vi "PH_BlackBox.PC Write PSDB.vi"(0 "i ref in":refnum<vi>, 5 "error IO":errorcluster) -> (14 "i ref out":refnum<vi>, 19 "error out":errorcluster)   [LabVIEW 2014, in "PH_BlackBox.lvlib"]
doc: "This is the proc case which writes data to the PHELIX shot data base."
uses:
  PH_BlackBox.lvlib
  PH_Basics/PH_PSDBWriter/PH_PSDBWriter.lvlib
  PH_Basics/PH_StatusHandler/PH_StatusHandler.lvlib
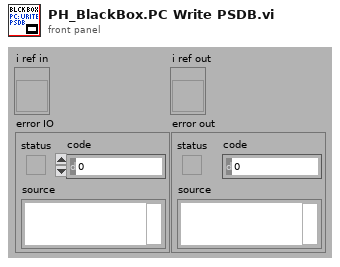
[diagram p1: front panel]
types:
  T1 = typedef "PH_BlackBox.lvlib/PH_BlackBox.i attribute.ctl" = cluster{"BB Remote Controlled?":bool, "GUI Refs":T2, "Position IN":T3, "Position OUT":T3, "BB Remote Controlled by other Instance?":bool, "Recipient":string, "Number":i32, "Caption Move":string, "Caption Out":string, "Caption In":string}
  T2 = typedef "PH_BlackBox.lvlib/PH_BlackBox.GUI Refs.ctl" = cluster{"MOVE IN":refnum<vi>, "MOVE":refnum<vi>, "IN":refnum<vi>, "OUT":refnum<vi>, "REMOTE":refnum<vi>, "GUI-Knob Move":refnum<vi>, "GUI-Knob Move in":refnum<vi>, "POWER ON":refnum<vi>, "Delete":refnum<vi>, "Function Textfield":refnum<vi>}
  T3 = typedef "PH_StatusHandler.lvlib/PH_StatusHandler.Status.ctl" = i16
  T4 = typedef "PH_PSDBWriter.lvlib/PH_PSDBWriter.String dataset.ctl" = cluster{"name":string, "data":string, "unit":string}
  T5 = typedef "PH_PSDBWriter.lvlib/PH_PSDBWriter.PSDB Dataset.ctl" = cluster{"Version":i32, "2D data Input":T6[], "Boolean Input":T8[], "Image Input":T9[], "Numeric Input":T11[], "String Input":T4[]}
  T6 = typedef "PH_PSDBWriter.lvlib/PH_PSDBWriter.2D dataset.ctl" = cluster{"name":string, "data":dbl[][], "axis description":T7}
  T7 = typedef "PSDB.lvlib/PSDB_AxisDescription.ctl" = cluster{"x axis label":string, "y axis label":string, "x axis unit":string, "y axis unit":string}
  T8 = typedef "PH_PSDBWriter.lvlib/PH_PSDBWriter.Boolean dataset.ctl" = cluster{"name":string, "data":bool, "unit":string}
  T9 = typedef "PH_PSDBWriter.lvlib/PH_PSDBWriter.Image dataset.ctl" = cluster{"name":string, "data":T10, "unit":string}
  T10 = typedef "IMAQ Image.ctl" = refnum<image>
  T11 = typedef "PH_PSDBWriter.lvlib/PH_PSDBWriter.Numeric dataset.ctl" = cluster{"name":string, "data":dbl, "unit":string}
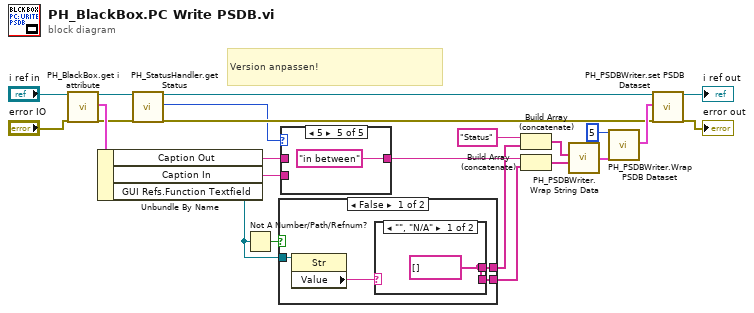
[diagram p0: block diagram]
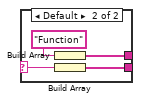
[diagram p2: hidden frame]
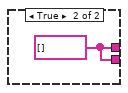
[diagram p3: hidden frame]
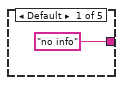
[diagram p4: hidden frame]
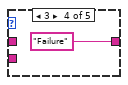
[diagram p7: hidden frame]
diagram:
  # "Version anpassen!"
  n1 = call "PH_BlackBox.get i attribute.vi"("i ref in"="i ref in", "error in (no error)"="error IO") -> ("i ref out"=w3:refnum<vi>, "i attribute"=w23:T1, "error out"=w22:errorcluster)  [unwired: 15 in]
  n2 = Unbundle By Name(w23) -> ("Caption Out"=w12:string, "Caption In"=w11:string, "GUI Refs.Function Textfield"=w7:refnum<vi>)
  n3 = call "PH_StatusHandler.get Status.vi"("VI in"=w3, "error in"=w22) -> ("VI out"=w2:refnum<vi>, "Status"=w1:T3, "error out"=w4:errorcluster)  [unwired: 15 in]
  n4 = Not A Number/Path/Refnum?(number/path/refnum=w7) -> (NaN/Path/Refnum?=w8:bool)
  n5 = case shown="False" w8 {
    tunnel: w7 -> [w26 _]
    tunnel: [w25 w33] -> w6
    tunnel: [w24 w33] -> w5
    frame False {
      n6 = property class="Str"(reference=w26) -> ("Value"=w27:string)  [unwired: 1 in, 2 out]
      n7 = case shown="\"\", \"N/A\"" w27 {
        selector: w27 -> [_ w32]
        tunnel: [w28 w30] -> w24
        tunnel: [w28 w29] -> w25
        frame "", "N/A" {
          w28 = string[] []
        }
        frame Default {
          n8 = Build Array("Function" ("Caption In")) -> (w29:string[])
          n9 = Build Array(w32) -> (w30:string[])
        }
      }
    }
    frame True {
      w33 = string[] []
    }
  }
  n10 = case shown="5" w1 {
    tunnel: w12 -> [_ w35 _ _ _]
    tunnel: w11 -> [_ _ w36 _ _]
    tunnel: ["no info" ("Caption In") w35 w36 "Failure" ("Caption In") "in between" ("Caption In")] -> w15
    frame Default {
    }
    frame 1 {
    }
    frame 2 {
    }
    frame 3 {
    }
    frame 5 {
    }
  }
  n11 = Build Array (concatenate)("Status" ("name"), w6) -> (w16:string[])
  n12 = Build Array (concatenate)(w15, w5) -> (w14:string[])
  n13 = call "PH_PSDBWriter.Wrap String Data.vi"("Data Array"=w14, "Name Array"=w16) -> ("PSDB String Data Array"=w13:T4[])  [unwired: 2 in]
  n14 = call "PH_PSDBWriter.Wrap PSDB Dataset.vi"("Version"=5, "String Input"=w13) -> ("PSDB Dataset"=w19:T5)  [unwired: 17 in]
  n15 = call "PH_PSDBWriter.set PSDB Dataset.vi"("VI in"=w2, "PSDB Dataset"=w19, "error in (no error)"=w4) -> ("VI out"=→"i ref out":refnum<vi>, "error out"=→"error out":errorcluster)  [unwired: 15 in]
